vi "PSD (Complex Multiply).vi"(0 "input 0":T1, 1 "reset":bool, 5 "input 1":T1, 7 "k":i16, 9 "input valid":bool) -> (4 "output":fxp<+/-,48,1>, 10 "output vliad":bool)   [LabVIEW 2018, in "NI PLL IP FPGA.lvlib"]
uses:
  NI PLL IP FPGA.lvlib
  <instrlib>/_niInstr/DSP/v1/Shared/Public/IQ Data.ctl
  <instrlib>/_niInstr/DSP/v1/FPGA/niInstr DSP v1 FPGA.lvlib
  <instrlib>/_niInstr/DSP/v1/Shared/niInstr DSP v1 Shared.lvlib
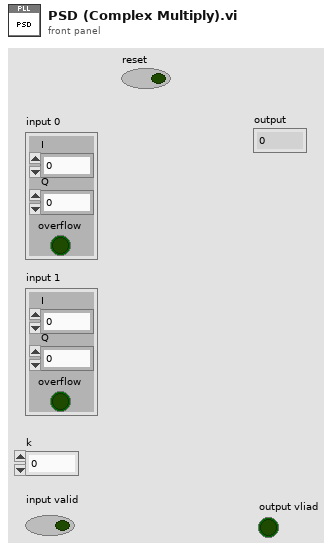
[diagram p1: front panel]
types:
  T1 = typedef "niInstr DSP v1 Shared.lvlib/IQ Data.ctl" = cluster{"I":fxp<+/-,18,1>, "Q":fxp<+/-,18,1>, "overflow":bool}
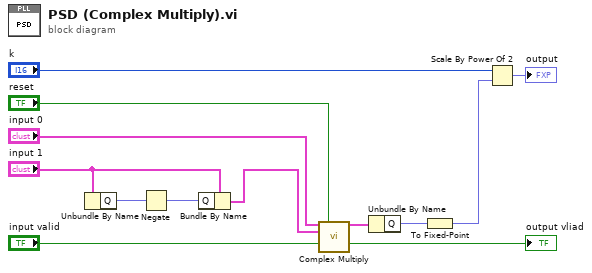
[diagram p0: block diagram]
diagram:
  n1 = Unbundle By Name("input 1") -> ("Q"=w4:fxp<+/-,18,1>)
  n2 = Negate(x=w4) -> (-x=w3:fxp<+/-,19,2>)
  n3 = Bundle By Name(cluster="input 1", "Q"=w3) -> (w1:T1)
  n4 = call <instrlib>:"Complex Multiply.vi"("IQ In 1"="input 0", "reset"="reset", "IQ In 2"=w1, "data valid in"="input valid") -> ("IQ Out"=w10:T1, "data valid out"=→"output vliad":bool)  [unwired: 10 in]
  n5 = Unbundle By Name(w10) -> ("Q"=w5:fxp<+/-,18,1>)
  n6 = To Fixed-Point(number=w5) -> (fixed-point=w9:fxp<+/-,48,1>)  [unwired: 1 in]
  n7 = Scale By Power Of 2(n="k", x=w9) -> (x*2^n=→"output":fxp<+/-,48,1>)
